vi "Adjust FP to Fit Controls.vi"(4 "Pane index (0)":i32, 6 "Error In":errorcluster, 8 "Controls & Decorations":refnum<vi>[](array[refnum]), 9 "VI ref":refnum<vi>) -> (0 "Error Out":errorcluster, 1 "PanelBounds":T1)   [LabVIEW 2018]
uses:
  <vilib>/Utility/miscctls.llb/LVRectTypeDef.ctl
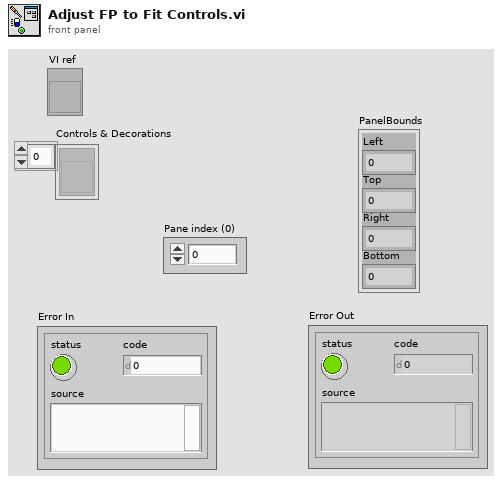
[diagram p1: front panel]
types:
  T1 = typedef "LVRectTypeDef.ctl" = cluster{"Left":i16, "Top":i16, "Right":i16, "Bottom":i16}
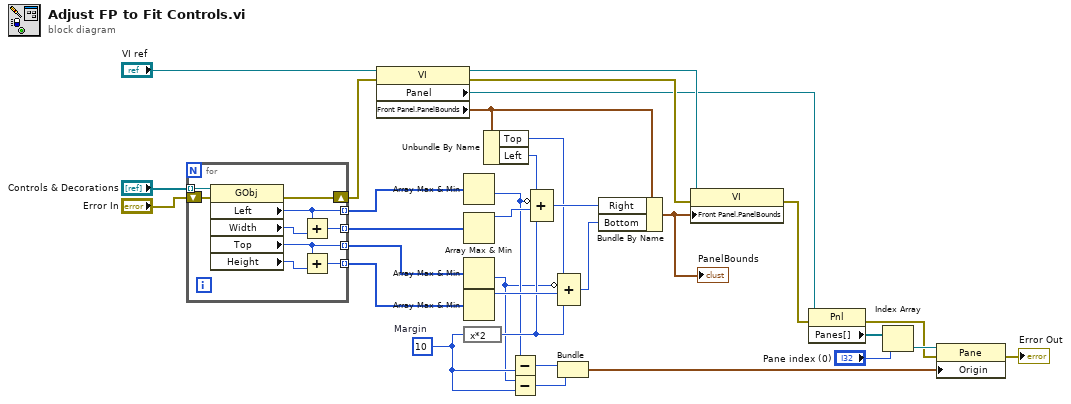
[diagram p0: block diagram]
diagram:
  w12 = 10  # Margin
  n1 = for {
    tunnel: "Controls & Decorations" -> [w35] mode=indexing
    tunnel: [w41] -> w30 mode=indexing
    tunnel: [w40] -> w29 mode=indexing
    tunnel: [w39] -> w27 mode=indexing
    tunnel: [w37] -> w28 mode=indexing
    shift-right: [w36] -> w7
    shift-left: "Error In" -> [w34]
    n2 = property class="GObj"(reference=w35, error in=w34) -> (error out=w36:errorcluster, "Left"=w41:i32, "Width"=w38:u32, "Top"=w37:i32, "Height"=w33:u32)  [unwired: 1 out]
    n3 = Add(x=w41, y=w38) -> (x+y=w40:u32)
    n4 = Add(x=w37, y=w33) -> (x+y=w39:u32)
  }
  n5 = property class="VI"(reference="VI ref", error in=w7) -> (reference out=w25:refnum<vi>, error out=w6:errorcluster, "Panel"=w5:refnum<vi>, "Front Panel.PanelBounds"=w26:T1)
  n6 = Array Max & Min(array=w30) -> (min value=w14:i32)  [unwired: 3 out]
  n7 = Array Max & Min(array=w29) -> (max value=w22:u32)  [unwired: 3 out]
  n8 = Array Max & Min(array=w28) -> (min value=w11:i32)  [unwired: 3 out]
  n9 = Array Max & Min(array=w27) -> (max value=w20:u32)  [unwired: 3 out]
  n10 = expression code="x*2"(w12) -> (w19:i32)
  n11 = Unbundle By Name(w26) -> ("Top"=w1:i16, "Left"=w23:i16)
  n12 = Subtract(x=w14, y=w12) -> (x-y=w13:i32)
  n13 = Subtract(x=w11, y=w12) -> (x-y=w10:i32)
  n14 = Compound Arithmetic op=ADD(w23, invert w14, w22, w19) -> (w21:u32)
  n15 = Compound Arithmetic op=ADD(w1, invert w11, w20, w19) -> (w18:u32)
  n16 = Bundle(w13, w10) -> (w9:cluster{i32, i32})  [unwired: 1 in]
  n17 = Bundle By Name(cluster=w26, "Right"=w21, "Bottom"=w18) -> (w24:T1)
  "PanelBounds" <- w24
  n18 = property class="VI"(reference=w25, error in=w6, "Front Panel.PanelBounds"=w24) -> (error out=w4:errorcluster)  [unwired: 1 out]
  n19 = property class="Pnl"(reference=w5, error in=w4) -> (error out=w3:errorcluster, "Panes[]"=w17:refnum<vi>[])  [unwired: 1 out]
  n20 = Index Array(array=w17, index="Pane index (0)") -> (element=w15:refnum<vi>)
  n21 = property class="Pane"(reference=w15, error in=w3, "Origin"=w9) -> (error out=→"Error Out":errorcluster)  [unwired: 1 out]
